vi "Read Access Token.vi"(8 "error in":errorcluster, 10 "password":string, 11 "username":string) -> (0 "error out":errorcluster, 2 "token":string)   [LabVIEW 2013, in "Spark API.lvlib"]
uses:
  Spark API.lvlib
  <vilib>/Utility/error.llb/Error Cluster From Error Code.vi
  <vilib>/ErrorRing/Error Ring.xnode
  <vilib>/httpClient/LabVIEWHTTPClient.lvlib
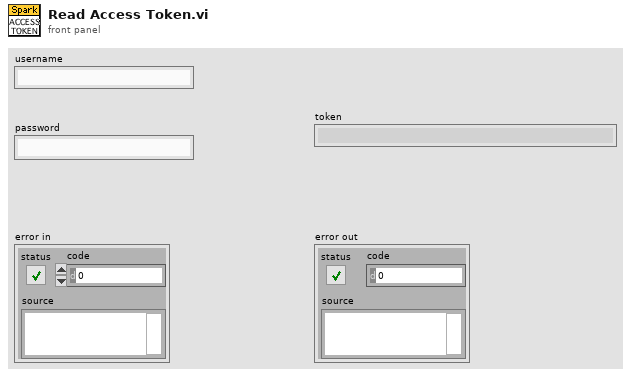
[diagram p1: front panel]
types:
  T1 = cluster{"token":string, "expires_at":string, "client":string}[]
  T2 = typedef "LabVIEWHTTPClient.lvlib/ClientHandle.ctl" = refnum<k1>
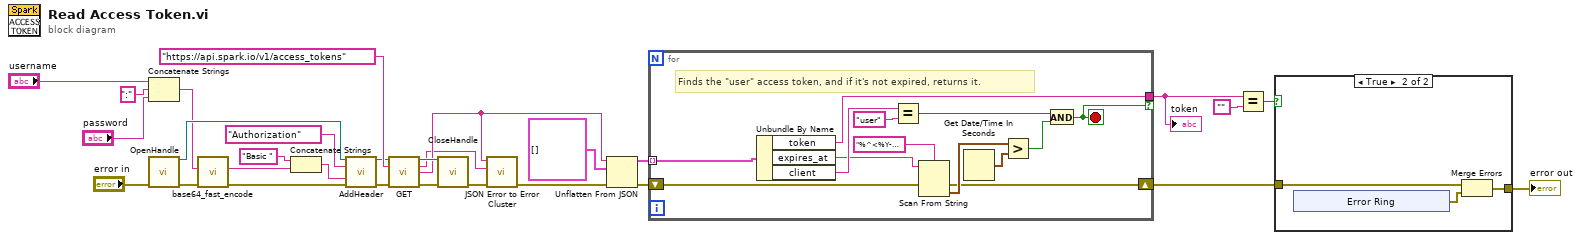
[diagram p0: block diagram]
diagram:
  n1 = Concatenate Strings("username", ":" ("string"), "password") -> (w17:string)
  n2 = call <vilib>:"OpenHandle.vi"("error in (no error)"="error in") -> ("client handle out"=w26:T2, "error out"=w22:errorcluster)  [unwired: 13 in]
  n3 = call "base64_fast_encode.vi"("error in (no error)"=w22, "string in (not encoded)"=w17) -> ("error out"=w23:errorcluster, "string out (base64-encoded)"=w15:string)  [unwired: 8 in]
  n4 = Concatenate Strings("Basic " ("string"), w15) -> (w16:string)
  n5 = call <vilib>:"AddHeader.vi"("client handle"=w26, "header"="Authorization", "value"=w16, "error in (no error)"=w23) -> ("client handle out"=w25:T2, "error out"=w27:errorcluster)  [unwired: 10 in]
  n6 = call <vilib>:"GET.vi"("client handle"=w25, "url"="https://api.spark.io/v1/access_tokens", "error in (no error)"=w27) -> ("client handle out"=w5:T2, "headers"=w1:string, "body"=w2:string, "error out"=w12:errorcluster)  [unwired: 9 in]
  n7 = call <vilib>:"CloseHandle.vi"("client handle"=w5, "error in (no error)"=w12) -> ("error out"=w4:errorcluster)  [unwired: 13 in]
  n8 = call "JSON Error to Error Cluster.vi"("error in (no error)"=w4, "headers"=w1, "JSON string"=w2) -> ("error out"=w3:errorcluster)  [unwired: 8 in]
  n9 = Unflatten From JSON(JSON string=w2, type and defaults=T1 [], error in (no error)=w3) -> (value=w13:T1, error out=w11:errorcluster)  [unwired: 4 in]
  n10 = for {
    tunnel: w13 -> [w42] mode=indexing
    tunnel: [w39] -> w10 if=w32
    shift-right: [w30] -> w8
    shift-left: w11 -> [w31]
    stop <- w32 stop-if-true
    # "Finds the \"user\" access token, and if it's not expired, returns it."
    n11 = Unbundle By Name(w42) -> ("token"=w39:string, "expires_at"=w37:string, "client"=w41:string)
    n12 = Equal?(x=w41, y="user") -> (x = y?=w33:bool)
    n13 = Scan From String(format string="%^<%Y-%m-%dT%H:%M:%S%3uZ>T", input string=w37, error in=w31) -> (error out=w30:errorcluster, output 1=w36:timestamp)  [unwired: 2 in, 2 out]
    n14 = Get Date/Time In Seconds() -> (seconds since 1Jan1904=w35:timestamp)
    n15 = Greater?(x=w36, y=w35) -> (0:w34:bool)
    n16 = And(x=w33, y=w34) -> (x .and. y?=w32:bool)
  }
  "token" <- w10
  n17 = Equal?(x=w10, y="") -> (x = y?=w6:bool)
  n18 = case shown="True" w6 {
    tunnel: w8 -> [w43 w45]
    tunnel: [w43 w44] -> w7
    frame False {
    }
    frame True {
      n19 = xnode "Error Ring"() -> ("error out"=w46:errorcluster)
      n20 = Merge Errors(w45, w46) -> (w44:errorcluster)
    }
  }
  "error out" <- w7
